vi "Read Channel Array.vi"(8 "error in (no error)":errorcluster, 11 "CIFCorePlugin in":refnum<class "CIFCorePlugin.lvclass">) -> (0 "error out":errorcluster, 2 "Channel Array":refnum<class "CIFChannels.lvclass">[](array[class]), 3 "CIFCorePlugin out":refnum<class "CIFCorePlugin.lvclass">)   [LabVIEW 2021, in "CIFCorePlugin.lvclass"]
uses:
  CIFCorePlugin.lvclass
  CIFCorePlugin.lvclass/CIFCorePlugin.ctl
  Channels/CIFChannelMng/CIFChannelMng.lvclass
  Channels/CIFChannels/CIFChannels.lvclass
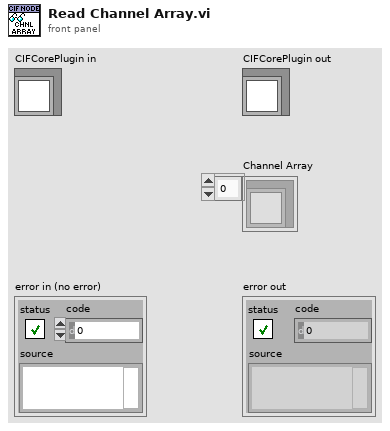
[diagram p1: front panel]
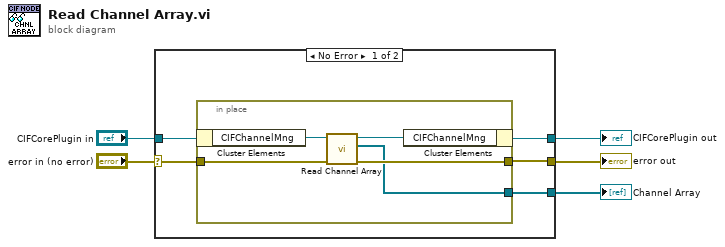
[diagram p0: block diagram]
diagram:
  n1 = case shown="No Error" "error in (no error)" {
    selector: "error in (no error)" -> [w8 w16]
    tunnel: [w7 w16] -> w3
    tunnel: [w9 w17] -> w2
    tunnel: "CIFCorePlugin in" -> [w10 w17]
    tunnel: [w6 _] -> w1
    frame No Error {
      n2 = in-place {
        in-place-border: w8 -> [w14]
        in-place-border: [w12] -> w7
        in-place-border: [w11] -> w6
        n3 = in-place-cluster #1(w10) -> ("CIFChannelMng"=w15:refnum<class "CIFChannelMng.lvclass">)
        n4 = call "Read Channel Array.vi"("error in (no error)"=w14, "CIFChannelMng in"=w15) -> ("error out"=w12:errorcluster, "Channel Array"=w11:refnum<class "CIFChannels.lvclass">[], "CIFChannelMng out"=w13:refnum<class "CIFChannelMng.lvclass">)  [unwired: 7 in]
        n5 = in-place-cluster #1("CIFChannelMng"=w13) -> (w9:refnum<class "CIFCorePlugin.lvclass">)
      }
    }
    frame Error {
    }
  }
  "error out" <- w3
  "CIFCorePlugin out" <- w2
  "Channel Array" <- w1
